vi "Command_AnalogOutput_v2.vi"() -> ()   [LabVIEW 2025]
uses:
  <vilib>/DAQmx/write.llb/DAQmx Write (Analog 1D DBL NChan 1Samp).vi
  <vilib>/DAQmx/create/channels.llb/DAQmx Create Channel (AO-Voltage-Basic).vi
  <vilib>/DAQmx/miscellaneous.llb/DAQmx Fill In Error Info.vi
  <resource>/objmgr/daqmx.rc
panel:
  in  "PURGE\nSOLENOID":bool
  out "error out":errorcluster
  in  "Needle Valve Voltage":dbl(slide) scale=-2.0..2.0
  in  "SOLENOID\nON/OFF":bool
  in  "IGNITION":bool
  in  "stop":bool
  # "Control Pannel"
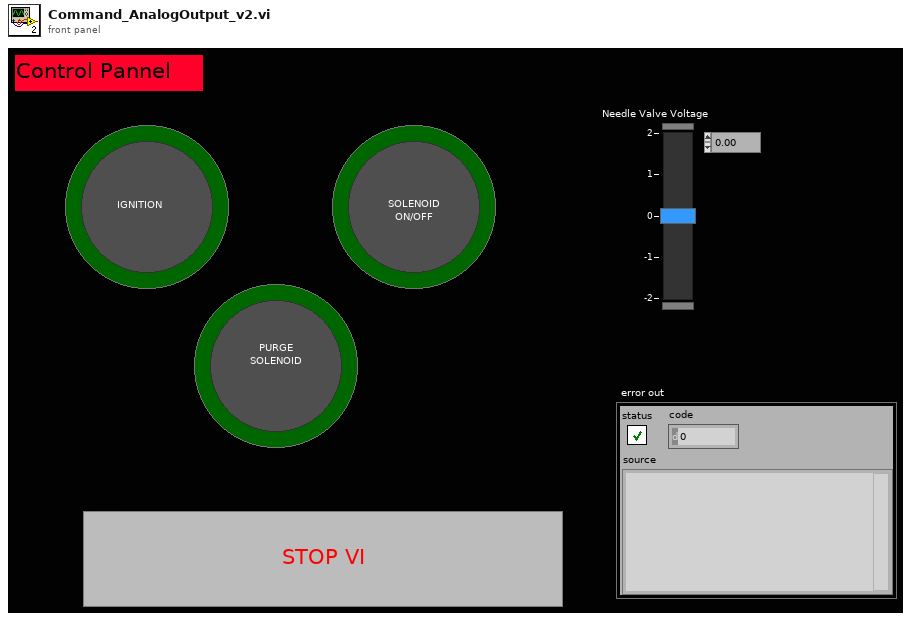
[diagram p1: front panel]
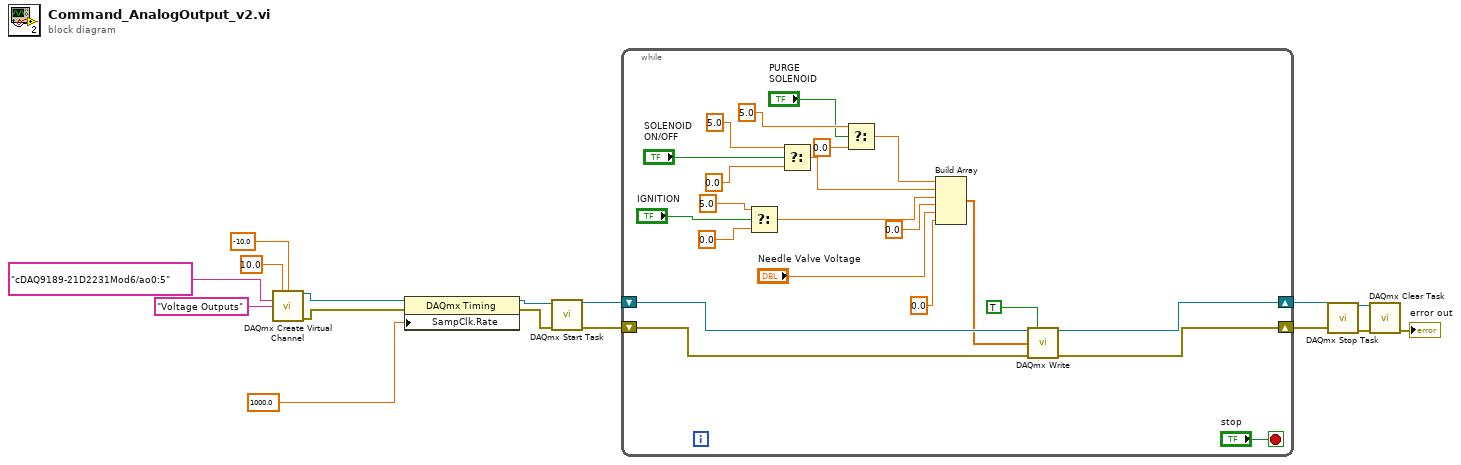
[diagram p0: block diagram]
diagram:
  n1 = call-poly <vilib>:"DAQmx Create Virtual Channel.vi"("maximum value"=10.0, "minimum value"=-10.0, "physical channels"="cDAQ9189-21D2231Mod6/ao0:5", "name to assign"="Voltage Outputs") -> ("task out"=w12:refnum<k21>, "error out"=w11:errorcluster)  [unwired: 10 in]
  n2 = property class="DAQmx Timing"(reference=w12, error in=w11, "SampClk.Rate"=1000.0) -> (reference out=w9:refnum<k21>, error out=w8:errorcluster)
  n3 = call <vilib>:"DAQmx Start Task.vi"("task/channels in"=w9, "error in"=w8) -> ("task out"=w7:refnum<k21>, "error out"=w6:errorcluster)  [unwired: 12 in]
  n4 = while {
    shift-right: [w35] -> w3
    shift-left: w7 -> [w37]
    shift-right: [w34] -> w2
    shift-left: w6 -> [w36]
    stop <- "stop" stop-if-true
    n5 = Select(t=5.0, s="IGNITION", f=0.0) -> (s? t:f=w30:dbl)
    n6 = Select(t=5.0, s="SOLENOID\nON/OFF", f=0.0 ("element")) -> (s? t:f=w25:dbl)
    n7 = Select(t=5.0 ("element"), s="PURGE\nSOLENOID", f=0.0 ("element")) -> (s? t:f=w17:dbl)
    n8 = Build Array(w17, w25, w30, 0.0 ("element"), "Needle Valve Voltage", 0.0 ("element")) -> (w22:dbl[])
    n9 = call-poly <vilib>:"DAQmx Write.vi"("task/channels in"=w37, "auto start"=TRUE, "data"=w22, "error in"=w36) -> ("task out"=w35:refnum<k21>, "error out"=w34:errorcluster)  [unwired: 9 in, 1 out]
  }
  n10 = call <vilib>:"DAQmx Stop Task.vi"("task/channels in"=w3, "error in"=w2) -> ("task out"=w4:refnum<k21>, "error out"=w5:errorcluster)  [unwired: 12 in]
  n11 = call <vilib>:"DAQmx Clear Task.vi"("task in"=w4, "error in"=w5) -> ("error out"=→"error out":errorcluster)  [unwired: 13 in]
